vi "实验车型选择比例 (子VI).vi"(10 "SG14百分比":dbl, 11 "D1":dbl) -> (3 "数值":dbl)   [LabVIEW 2016]
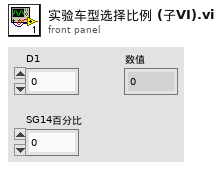
[diagram p1: front panel]
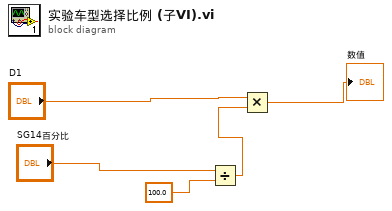
[diagram p0: block diagram]
diagram:
  n1 = Divide(x="SG14百分比", y=100.0) -> (x/y=w4:dbl)
  n2 = Multiply(x="D1", y=w4) -> (x*y=→"数值":dbl)
